vi "Generate Waveform.vi"(8 "error in":errorcluster, 11 "Generator in":refnum<class "Generador.lvclass">) -> (0 "error out":errorcluster, 2 "Waveform":waveform(dbl), 3 "Generator out":refnum<class "Generador.lvclass">)   [LabVIEW 2020, in "FGen.lvlib" / "Generador.lvclass"]
uses:
  Generador.lvclass
  Generador.lvclass/Generador.ctl
  Get offset.vi
  Get signal type.vi
  Get frequency.vi
  Get amplitude.vi
  Get phase.vi
  Get sampling info.vi
  Get square wave duty cycle (%).vi
  <vilib>/measure/NI_MABase.lvlib
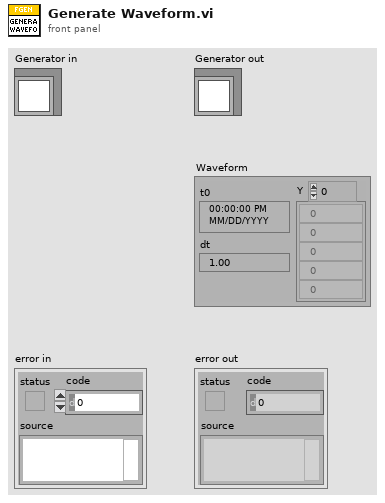
[diagram p1: front panel]
types:
  T1 = enum16{"Sine Wave", "Triangle Wave", "Square Wave", "Sawtooth Wave"}
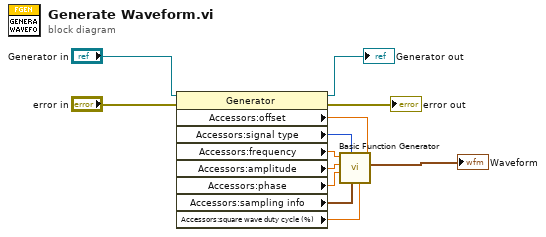
[diagram p0: block diagram]
diagram:
  n1 = property class="Generator"(reference="Generator in", error in="error in") -> (reference out=→"Generator out":refnum<class "Generador.lvclass">, error out=→"error out":errorcluster, "Accessors:offset"=w8:dbl, "Accessors:signal type"=w7:T1, "Accessors:frequency"=w6:dbl, "Accessors:amplitude"=w5:dbl, "Accessors:phase"=w4:dbl, "Accessors:sampling info"=w3:cluster{"Fs":dbl, "#s":dbl}, "Accessors:square wave duty cycle (%)"=w2:dbl)
  n2 = call <vilib>:"Basic Function Generator.vi"("offset"=w8, "square wave duty cycle (%)"=w2, "sampling info"=w3, "signal type"=w7, "phase"=w4, "amplitude"=w5, "frequency"=w6) -> ("signal out"=→"Waveform":waveform(dbl))  [unwired: 2 in, 2 out]
